vi "Color Byte Swap.vi"(11 "Image Pixels (U32) in":u32[](array[numeric])) -> (3 "Images Pixels Out":u32[](array[numeric]))   [LabVIEW 2013]
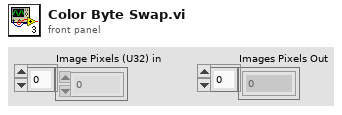
[diagram p1: front panel]
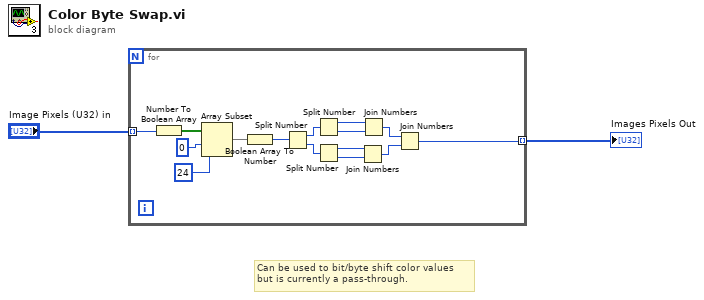
[diagram p0: block diagram]
diagram:
  # "Can be used to bit/byte shift color values\nbut is currently a pass-through."
  n1 = for {
    tunnel: "Image Pixels (U32) in" -> [w17] mode=indexing
    tunnel: [w5] -> w2 mode=indexing
    n2 = Number To Boolean Array(number=w17) -> (Boolean array=w16:bool[])
    n3 = Array Subset(array=w16, index=0, length=24) -> (w13:bool[])
    n4 = Boolean Array To Number(Boolean array=w13) -> (number=w12:u32)
    n5 = Split Number(x=w12) -> (hi(x)=w10:u16, lo(x)=w11:u16)
    n6 = Split Number(x=w10) -> (hi(x)=w7:u8, lo(x)=w8:u8)
    n7 = Split Number(x=w11) -> (hi(x)=w3:u8, lo(x)=w4:u8)
    n8 = Join Numbers(hi=w3, lo=w4) -> ((hi.lo)=w6:u16)
    n9 = Join Numbers(hi=w7, lo=w8) -> ((hi.lo)=w9:u16)
    n10 = Join Numbers(hi=w9, lo=w6) -> ((hi.lo)=w5:u32)
  }
  "Images Pixels Out" <- w2
